vi "Adv_WriteLightFieldProperty.vi"(8 "error in (no error)":errorcluster, 9 "value":refnum<k24>, 10 "setting":string, 11 "LightField Automation in":refnum<class "LightField Automation.lvclass">) -> (0 "error out":errorcluster, 3 "LightField Automation out":refnum<class "LightField Automation.lvclass">)   [LabVIEW 2013, in "LightField Automation.lvclass"]
uses:
  LightField Automation.lvclass
  LightField Automation.lvclass/LightField Automation.ctl
  C:/Program Files/Princeton Instruments/LightField/AddInViews/PrincetonInstruments.LightFieldViewV3.dll
  Program Files/Princeton Instruments/LightField/AddInViews/PrincetonInstruments.LightFieldViewV3.dll
  <vilib>/Utility/error.llb/DialogType.ctl
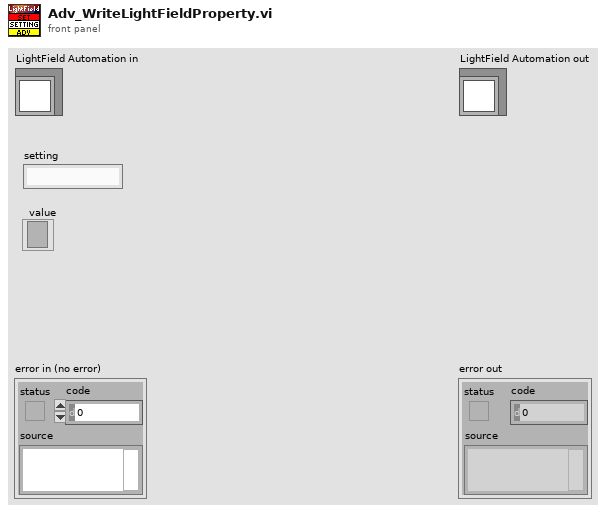
[diagram p1: front panel]
types:
  T1 = typedef "DialogType.ctl" = u16
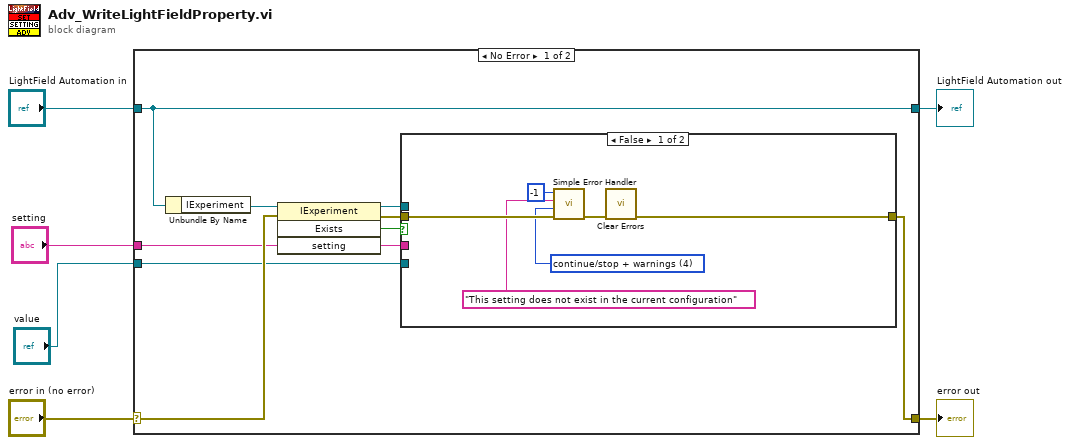
[diagram p0: block diagram]
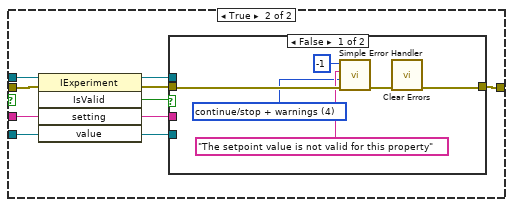
[diagram p2: hidden frame]
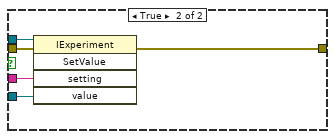
[diagram p3: hidden frame]
diagram:
  n1 = case shown="No Error" "error in (no error)" {
    selector: "error in (no error)" -> [w12 w42]
    tunnel: [w15 w42] -> w5
    tunnel: [w14 w41] -> w3
    tunnel: "LightField Automation in" -> [w14 w41]
    tunnel: "setting" -> [w8 _]
    tunnel: "value" -> [w7 _]
    frame No Error {
      n2 = Unbundle By Name(w14) -> ("IExperiment"=w13:refnum<k24>)
      n3 = invoke class="IExperiment" method="Exists"(reference=w13, error in=w12, "setting"=w8) -> (reference out=w10:refnum<k24>, error out=w9:errorcluster, "Exists"=w11:bool)  [unwired: 1 in, 1 out]
      n4 = case shown="False" w11 {
        tunnel: [w17 w29] -> w15
        tunnel: w10 -> [_ w28]
        tunnel: w9 -> [w21 w27]
        tunnel: w8 -> [_ w23]
        tunnel: w7 -> [_ w22]
        frame False {
          w16 = T1 4 items=["no dialog", "OK message", "continue or stop message", "OK message + warnings", "continue/stop + warnings"] ("type of dialog (OK msg:1)")
          n5 = call <vilib>:"Simple Error Handler.vi"("error code (no error:0)"=-1, "error source (\" \")"="This setting does not exist in the current configuration" ("source"), "type of dialog (OK msg:1)"=w16, "error in (no error)"=w21) -> ("error out"=w18:errorcluster)  [unwired: 1 in, 4 out]
          n6 = call <vilib>:"Clear Errors.vi"("error in (no error)"=w18) -> ("error out"=w17:errorcluster)  [unwired: 6 in]
        }
        frame True {
          n7 = invoke class="IExperiment" method="IsValid"(reference=w28, error in=w27, "setting"=w23, "value"=w22) -> (reference out=w25:refnum<k24>, error out=w24:errorcluster, "IsValid"=w26:bool)  [unwired: 1 in, 2 out]
          n8 = case shown="False" w26 {
            tunnel: [w32 w40] -> w29
            tunnel: w25 -> [_ w39]
            tunnel: w24 -> [w33 w38]
            tunnel: w23 -> [_ w37]
            tunnel: w22 -> [_ w36]
            frame False {
              w30 = T1 4 items=["no dialog", "OK message", "continue or stop message", "OK message + warnings", "continue/stop + warnings"] ("type of dialog (OK msg:1)")
              n9 = call <vilib>:"Simple Error Handler.vi"("error code (no error:0)"=-1, "error source (\" \")"="The setpoint value is not valid for this property" ("source"), "type of dialog (OK msg:1)"=w30, "error in (no error)"=w33) -> ("error out"=w34:errorcluster)  [unwired: 1 in, 4 out]
              n10 = call <vilib>:"Clear Errors.vi"("error in (no error)"=w34) -> ("error out"=w32:errorcluster)  [unwired: 6 in]
            }
            frame True {
              n11 = invoke class="IExperiment" method="SetValue"(reference=w39, error in=w38, "setting"=w37, "value"=w36) -> (error out=w40:errorcluster)  [unwired: 1 in, 4 out]
            }
          }
        }
      }
    }
    frame Error {
    }
  }
  "error out" <- w5
  "LightField Automation out" <- w3
